vi "Get Data.vi"(8 "error in (no error)":errorcluster, 11 "Cap Bank Idot Measurement in":refnum<class "Cap Bank Idot Measurement.lvclass">) -> (0 "error out":errorcluster, 3 "Cap Bank Idot Measurement out":refnum<class "Cap Bank Idot Measurement.lvclass">)   [LabVIEW 2015, in "Cap Bank Idot Measurement.lvclass"]
uses:
  Cap Bank Idot Measurement.lvclass
  <vilib>/ActorFramework/Actor/Actor.lvclass/Actor.ctl
  Mag Lab Measure Controller Messages/Log Status Update Msg/Log Status Update Msg.lvclass/Log Status Update Msg.ctl
  <vilib>/ActorFramework/Message Enqueuer/Message Enqueuer.lvclass/Message Enqueuer.ctl
  Cap Bank Server Messages/Recieve Idot Result Msg/Recieve Idot Result Msg.lvclass/Recieve Idot Result Msg.ctl
  <vilib>/ActorFramework/Message Enqueuer/Enqueue.vi
  <vilib>/ActorFramework/Message Priority Queue/Priority Enqueue.vi
  Mag Lab Measure Controller Messages/Log Status Update Msg/Log Status Update Msg.lvclass
  Cap Bank Server Messages/Recieve Idot Result Msg/Recieve Idot Result Msg.lvclass
  <vilib>/ActorFramework/Actor/Actor.lvclass
  Mag Lab Error Handler/Mag Lab Error Handler.lvclass
  NI-DAQ/Mag Lab Measure/DAQmx Digitizer/DAQmx Digitizer.lvclass
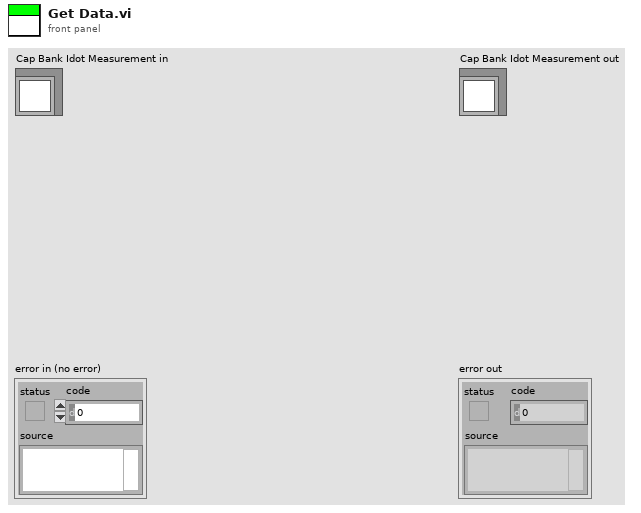
[diagram p1: front panel]
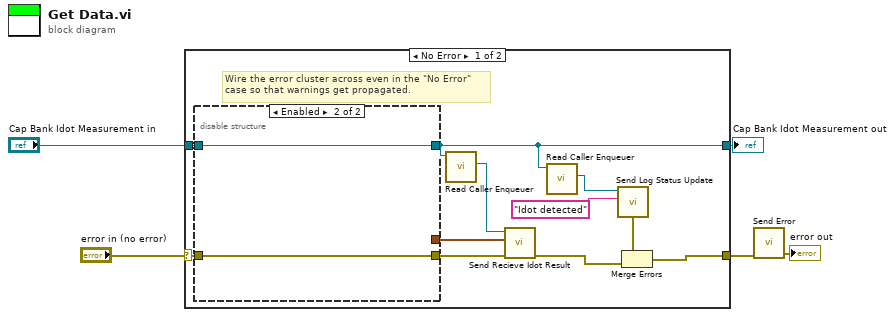
[diagram p0: block diagram]
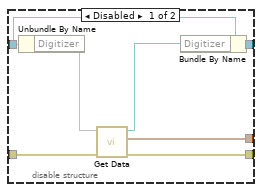
[diagram p2: hidden frame]
diagram:
  n1 = case shown="No Error" "error in (no error)" {
    selector: "error in (no error)" -> [w15 w27]
    tunnel: [w7 w27] -> w2
    tunnel: [w12 w26] -> w3
    tunnel: "Cap Bank Idot Measurement in" -> [w16 w26]
    frame No Error {
      # "Wire the error cluster across even in the \"No Error\"\ncase so that warnings get propagated."
      n2 = disable-structure shown="Enabled" {
        disable-tunnel: w16 -> [w23 w25]
        disable-tunnel: w15 -> [w20 w24]
        disable-tunnel: [w19 _] -> w13
        disable-tunnel: [w18 w25] -> w12
        disable-tunnel: [w17 w24] -> w8
        frame Disabled {
          n3 = Unbundle By Name(w23) -> ("Digitizer"=w22)
          n4 = call-dynamic "Get Data.vi"("error in (no error)"=w20, "DAQmx Digitizer in"=w22) -> ("error out"=w17:errorcluster, "data"=w19:waveform(dbl)[], "DAQmx Digitizer out"=w21:refnum<class "DAQmx Digitizer.lvclass">)  [unwired: 7 in]
          n5 = Bundle By Name(cluster=w23, "Digitizer"=w21) -> (w18:refnum<class "Cap Bank Idot Measurement.lvclass">)
        }
        frame Enabled {
        }
      }
      n6 = call <vilib>:"Read Caller Enqueuer.vi"("Actor"=w12) -> ("Caller Enqueuer"=w14:refnum<class "Message Enqueuer.lvclass">)  [unwired: 10 in]
      n7 = call "Send Recieve Idot Result.vi"("error in (no error)"=w8, "Idot data"=w13, "Message Enqueuer"=w14) -> ("error out"=w6:errorcluster)  [unwired: 7 in, 1 out]
      n8 = call <vilib>:"Read Caller Enqueuer.vi"("Actor"=w12) -> ("Caller Enqueuer"=w11:refnum<class "Message Enqueuer.lvclass">)  [unwired: 10 in]
      n9 = call "Send Log Status Update.vi"("Status"="Idot detected", "Message Enqueuer"=w11) -> ("error out"=w9:errorcluster)  [unwired: 8 in, 1 out]
      n10 = Merge Errors(w9, w6) -> (w7:errorcluster)
    }
    frame Error {
    }
  }
  "Cap Bank Idot Measurement out" <- w3
  n11 = call "Send Error.vi"("error in (no error)"=w2) -> ("error out"=→"error out":errorcluster)  [unwired: 9 in, 1 out]
